vi "Disconnect.vi"(8 "error in":errorcluster) -> (0 "error out":errorcluster)   [LabVIEW 2016, in "TCP.lvlib"]
uses:
  TCP.lvlib
  Support/Message Queue/Enqueue Message (Single).vi
  support/Message Queue/Message Queue.lvlib
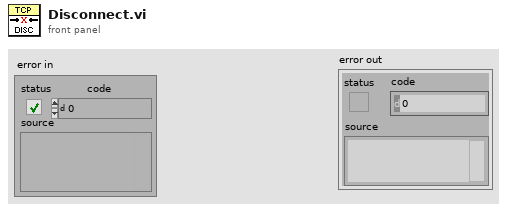
[diagram p1: front panel]
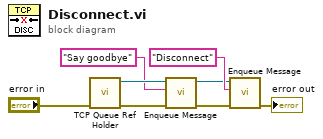
[diagram p0: block diagram]
diagram:
  n1 = call "TCP Queue Ref Holder.vi"("error in"="error in") -> ("error out"=w5:errorcluster, "Input Message Queue"=w3:refnum<queue>)  [unwired: 9 in]
  n2 = call-poly "Enqueue Message.vi"("error in (no error)"=w5, "Message"="Say goodbye", "Message Queue"=w3) -> ("error out"=w4:errorcluster, "dup Message Queue"=w2:refnum<queue>)  [unwired: 7 in]
  n3 = call-poly "Enqueue Message.vi"("error in (no error)"=w4, "Message"="Disconnect", "Message Queue"=w2) -> ("error out"=→"error out":errorcluster)  [unwired: 7 in, 1 out]
